vi "Interface.vi"() -> ()   [LabVIEW 2018]
uses:
  Readout Delay Charact/Readout Charact.lvclass
  CCDCamera/CCDCamera.lvclass
  Interface/Interface.lvclass
  Cooler/Cooler.lvclass
  Sync Box/Sync Box.lvclass
  State Machine/State Machine.lvclass
panel:
  in  "Trigger":u16(ring) items=["Internal", "External", "N/A", "N/A", "N/A", "N/A", "External Start"]
  in  "Vertical Clock  Amplitude":u8(ring) items=["Normal", "+1", "+2", "+3", "+4"]
  out "Readout Time (ms)":dbl=0.039386453333333335
  in  "Camera Setup":T1={"Image Name"="Image", "Image Path"="C:\\Users\\Cliente\\Desktop\\SPARC4_AC\\Imagens\\", "# Images"=0, "Exposure Time"=0.0, "Pre-amp gain"=0, "Readout Rate"=0, "Vertical Shift Speed"=3, "Acquisition Mode"=1, "Read Mode"=4, "EM Mode"=0, "EM Gain"=2, "Shutter Mode"=2, "Shutter TTL"=0, "Time to open shutter"=50, "Time to close shutter"=50, "Vertical Binning"=1, "Horizontal Binning"=1, "Initial Line"=1, "Initial Cloumn"=1, "Final Line"=1024, "Final Column"=1024, "Cooler ON/OFF"=0, "Set temperature"=20, "Number of exp"=0, "Exposições realizadas"=0, "Kinetic Serie Length"=0, "Number of Accumulations"=0, "Kinetic Cycle Time"=0, "Frame Transfer"=FALSE, "Vertical Clock  Amplitude"=0, "Trigger"=0} {"Trigger" items=["Internal", "External", "N/A", "N/A", "N/A", "N/A", "External Start"]; "Vertical Clock  Amplitude" items=["Normal", "+1", "+2", "+3", "+4"]; "Set temperature" min=0 max=0; "Cooler ON/OFF" items=["Cooler OFF", "Cooler ON"]; "Shutter TTL" items=["TTL Low", "TTl High"]; "Shutter Mode" items=["Fully Auto", "OPEN", "CLOSED"]; "EM Mode" items=["Electron Multiplying", "Conventional"]; "Read Mode" items=["Full Vertical Binning", "Multi-Track", "Random-track", "Single-Track", "Image"]; "Acquisition Mode" items=["N/A", "Single", "Accumulate", "Kinetic", "Fast Kinetic"]; "Vertical Shift Speed" items=["0.6", "1.13", "2.2", "4.33"]; "Readout Rate" items=["1 MHz", "10 MHz", "20 MHz", "30 MHz"]; "Pre-amp gain" items=["Gain 1", "Gain 2"]}
  in  "Frame Transfer":bool
  in  "Number of Accum.":u32=1 min=1
  in  "Kinetic Cycle Time":u32
  in  "Kinetic Series Length":u32=1 min=1
  out "String":string="#img      1st Time       2nd Time      3th Time      4th Time      5th Time\n------------------------------------------------------------------------\n"
  in  "Tempo de espera":u16=20
  out "Calculated Delay Series:":dbl
  in  "Address:":string="192.168.254.183"
  in  "Remote Port:":u32=2000
  in  "Stop Button":bool
  in  "Readout Charact in":refnum<class "Readout Charact.lvclass">
  in  "Vertical Binning":u16=1
  in  "Horizontal Binning":u16=1
  in  "Final Line":u16=1024
  in  "Final Column":u16=1024
  in  "Initial Cloumn":u16=1
  in  "Initial Line":u16=1
  in  "Time to open shutter":u16=50
  in  "Time to close shutter":u16=50
  in  "Shutter Mode":u8(ring)=2 items=["Fully Auto", "OPEN", "CLOSED"]
  in  "Shutter TTL":u8(ring) items=["TTL Low", "TTl High"]
  in  "Set temperature":i8=20 min=-120 max=20
  in  "Cooler ON/OFF":u16(ring) items=["Cooler OFF", "Cooler ON"]
  in  "EM Mode":u8(ring) items=["Electron Multiplying", "Conventional"]
  in  "EM Gain":u16=2 min=2 max=300
  in  "Pre-amp gain":u8(ring) items=["Gain 1", "Gain 2", "Gain 3"]
  in  "Readout Rate":u8(ring) items=["30 MHz", "20 MHz", "10 MHz", "  1 MHz"]
  in  "Vertical Shift Speed":u8(ring)=3 items=["0.6", "1.13", "2.2", "4.33"]
  in  "Acquisition Mode":u8(ring)=1 items=["N/A", "Single", "Accumulate", "Kinetic", "Fast Kinetic"]
  in  "Read Mode":u8(ring)=4 items=["Full Vertical Binning", "Multi-Track", "Random-track", "Single-Track", "Image"]
  in  "Image Name":string="CH1"
  out "Initialization":bool
  in  "Exposure Time":u32
  in  "# Images":u32=1 min=1
  out "Temperature":i16
  out "Exposing":bool
  out "% Acquired":dbl format="%#.2g"
  out "Exposições realizadas":u8(slide) max=1 scale=0.0..1.0
  in  "Abort":bool
  in  "Adquirir":bool
  in  "Stop Acq":bool
  in  "Pausar":bool
  in  "Image Path":string="C:\\Users\\observer\\Desktop\\SPARC4 Acquisition Control\\Imagens"
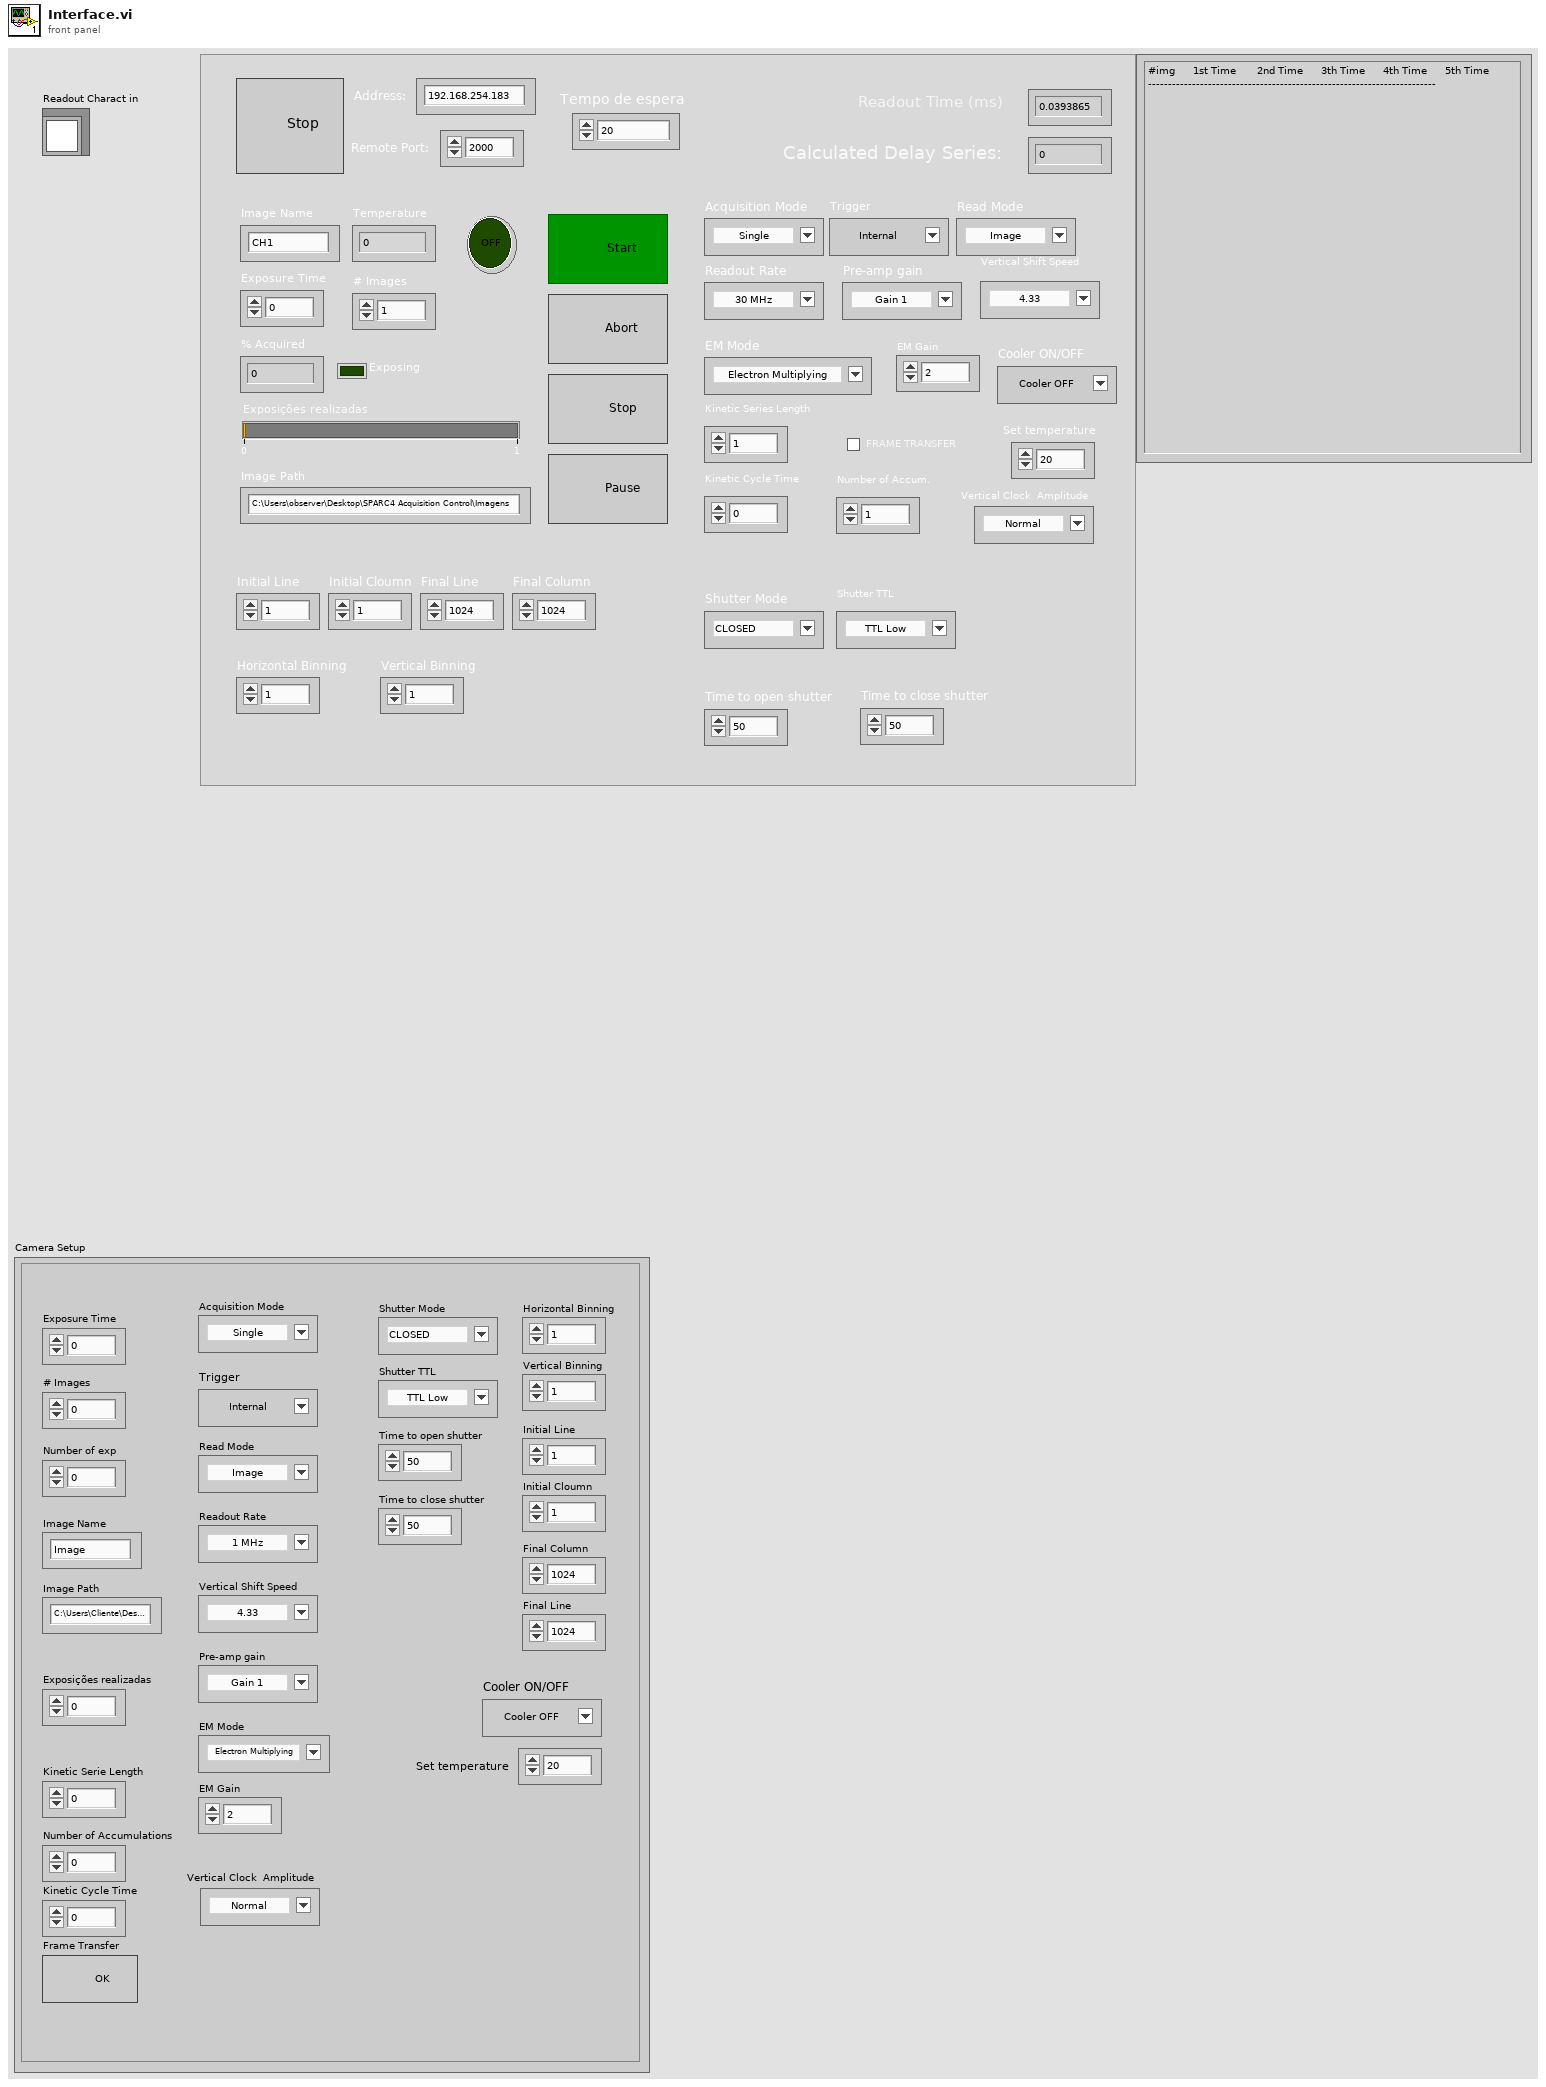
[diagram p1: front panel]
types:
  T1 = cluster{"Image Name":string, "Image Path":string, "# Images":u32, "Exposure Time":dbl, "Pre-amp gain":u8, "Readout Rate":u8, "Vertical Shift Speed":u8, "Acquisition Mode":u8, "Read Mode":u8, "EM Mode":u8, "EM Gain":u16, "Shutter Mode":u8, "Shutter TTL":u8, "Time to open shutter":u16, "Time to close shutter":u16, "Vertical Binning":u16, "Horizontal Binning":u16, "Initial Line":u16, "Initial Cloumn":u16, "Final Line":u16, "Final Column":u16, "Cooler ON/OFF":u16, "Set temperature":i8, "Number of exp":u32, "Exposições realizadas":u16, "Kinetic Serie Length":u32, "Number of Accumulations":u32, "Kinetic Cycle Time":u32, "Frame Transfer":bool, "Vertical Clock  Amplitude":u8, "Trigger":u16}
  T2 = cluster{"% Acquired":dbl, "Acquiring":bool, "Current Temperature":dbl, "Temperatue Status":string, "Min Temp":dbl, "Max Temp":dbl, "Exposições realizadas":u32, "Final Column":u16, "Final Line":u16}
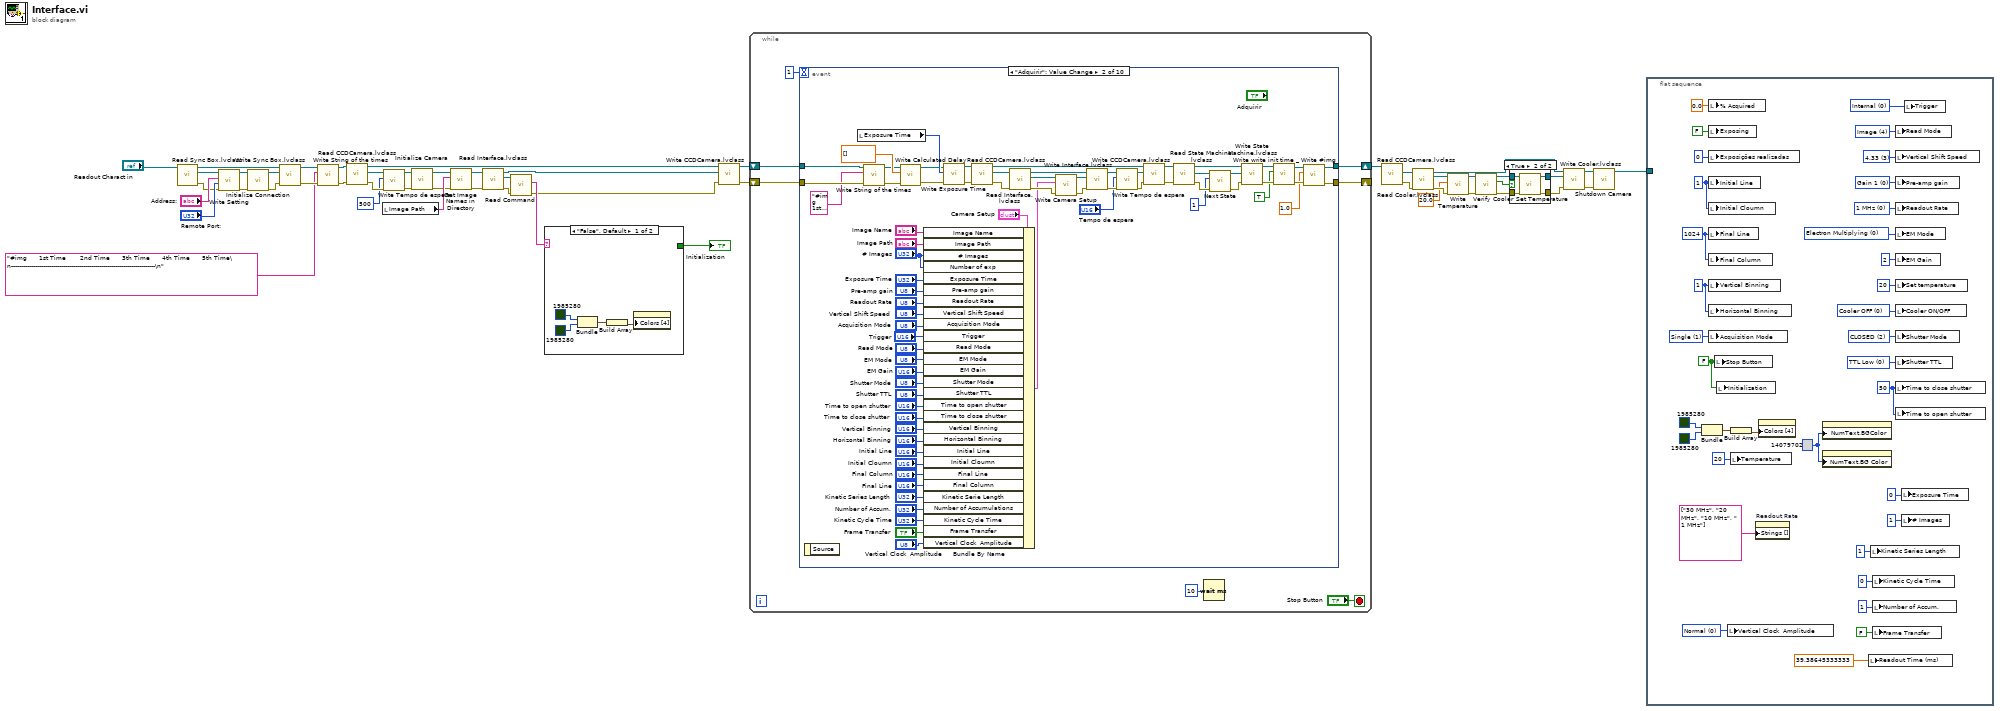
[diagram p0: block diagram]
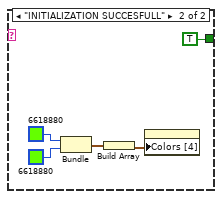
[diagram p2: hidden frame]
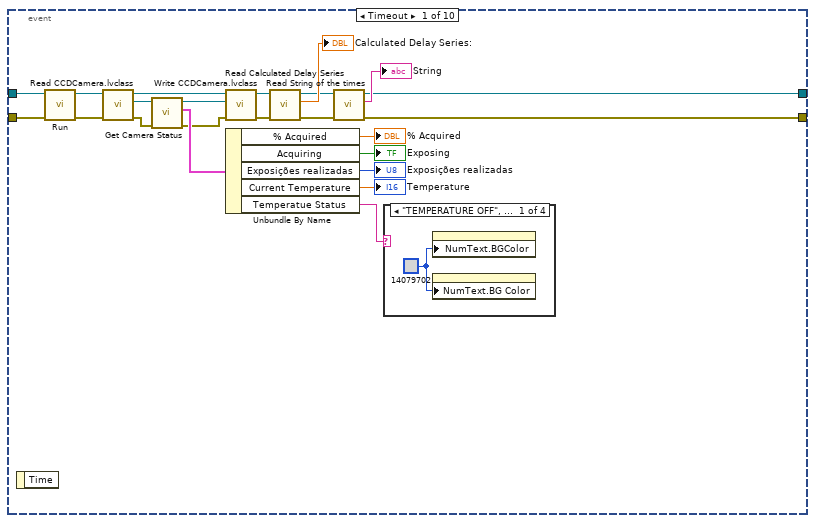
[diagram p4: hidden frame]
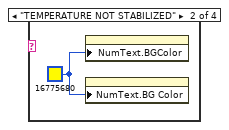
[diagram p5: hidden frame]
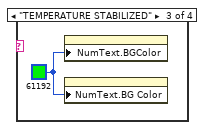
[diagram p6: hidden frame]
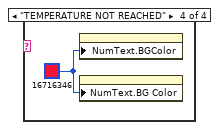
[diagram p7: hidden frame]
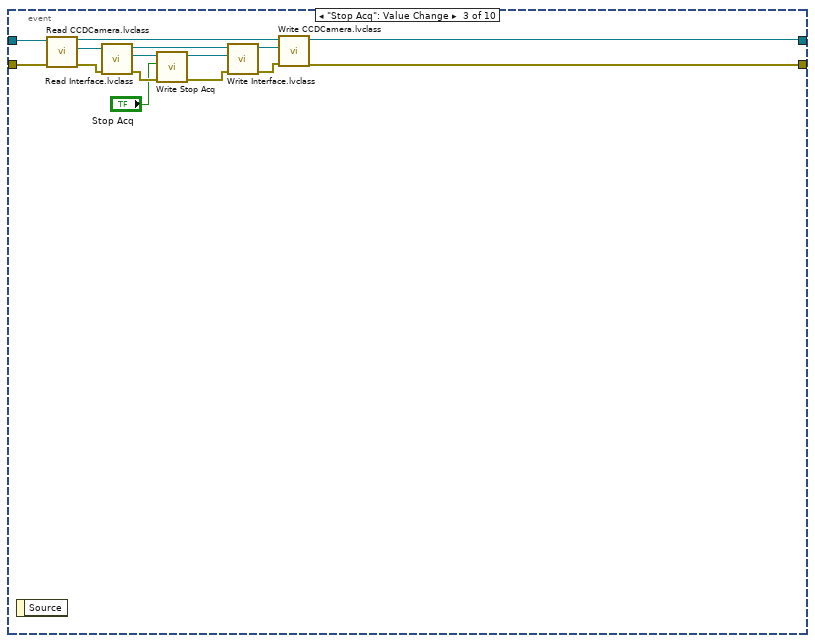
[diagram p8: hidden frame]
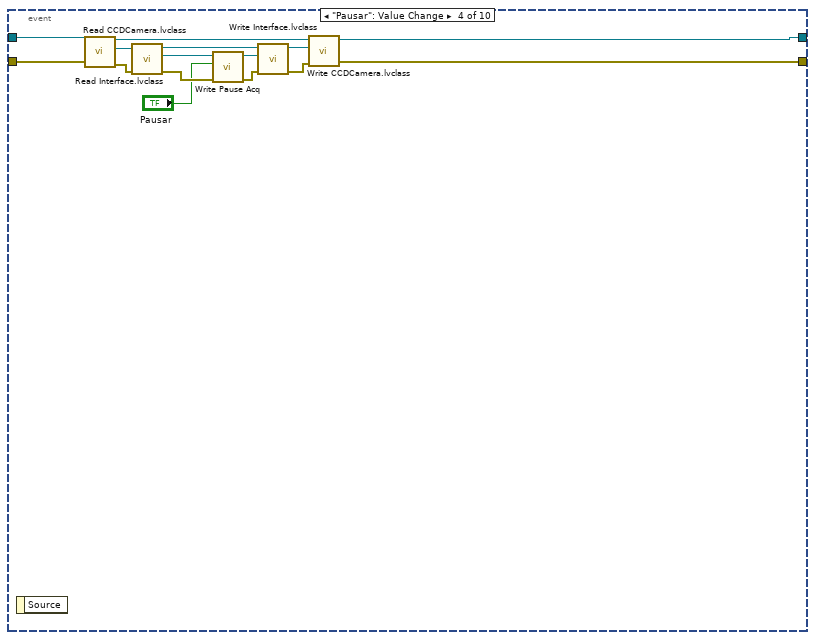
[diagram p9: hidden frame]
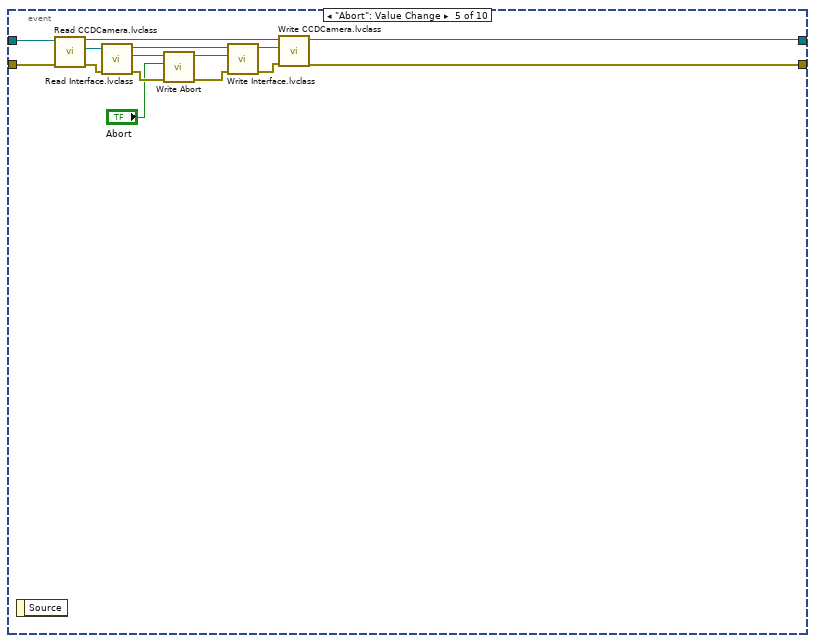
[diagram p10: hidden frame]
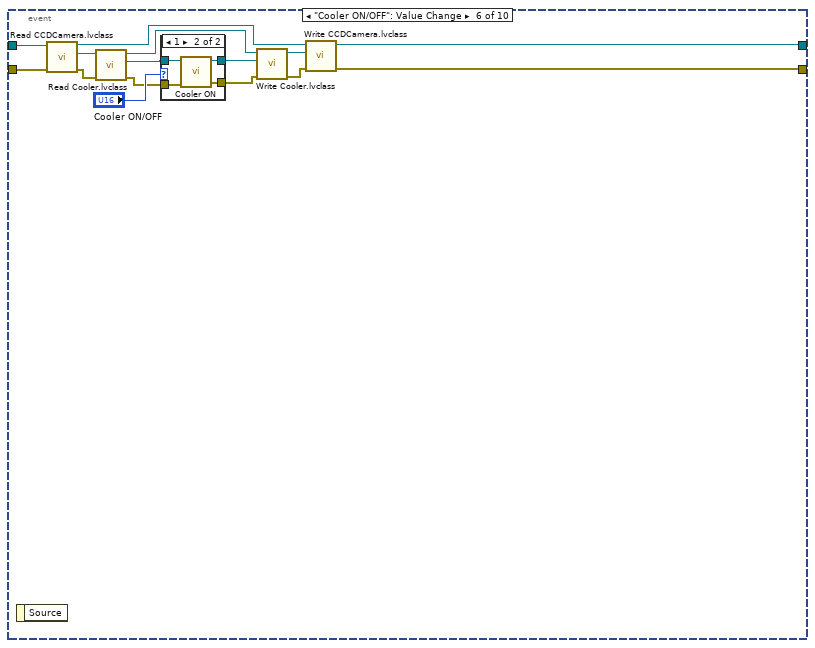
[diagram p11: hidden frame]
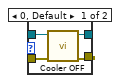
[diagram p12: hidden frame]
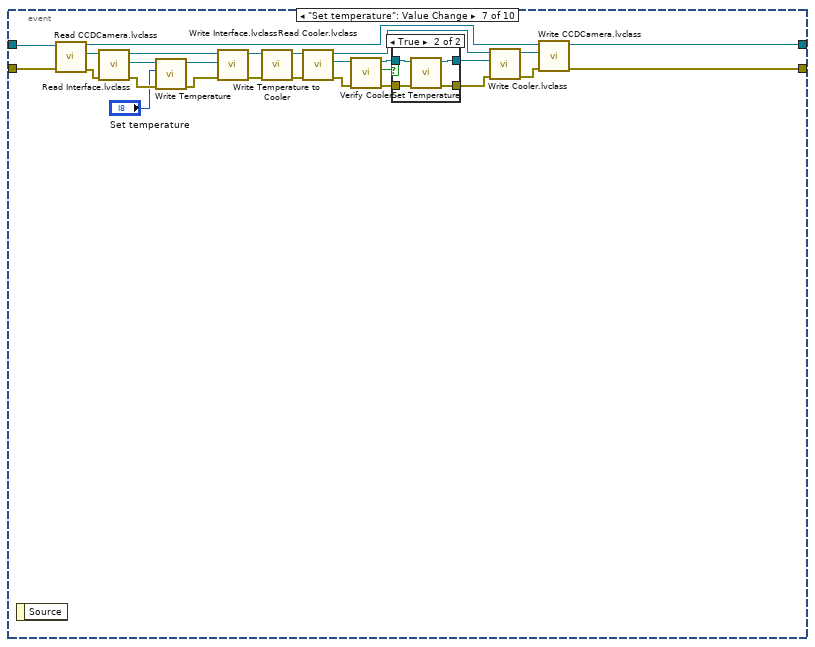
[diagram p13: hidden frame]
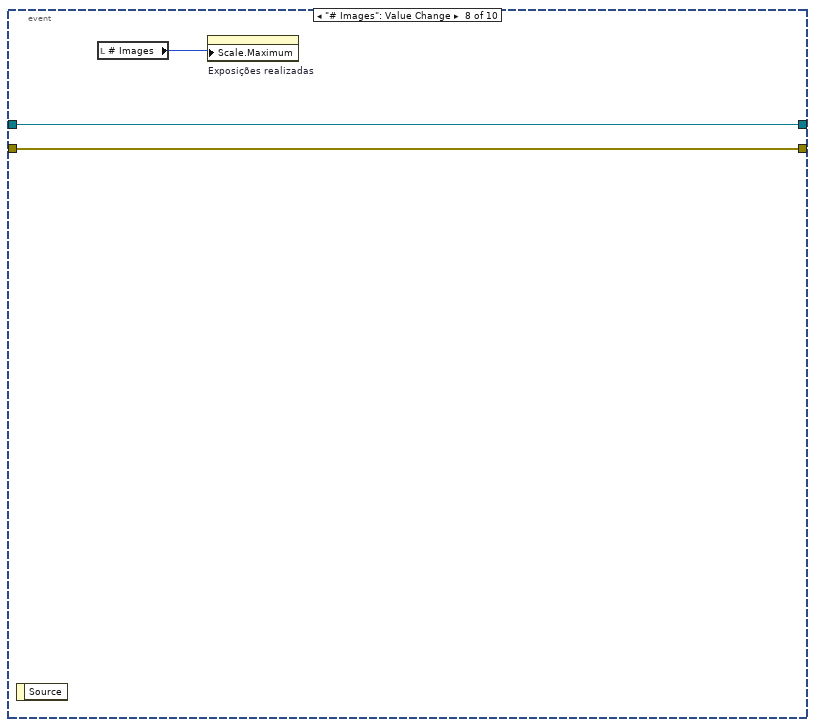
[diagram p15: hidden frame]
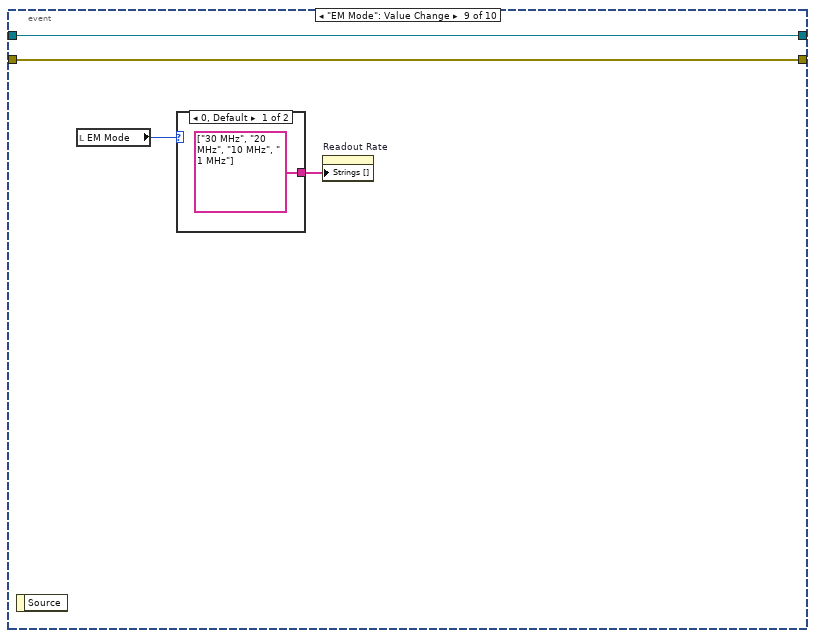
[diagram p16: hidden frame]
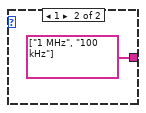
[diagram p17: hidden frame]
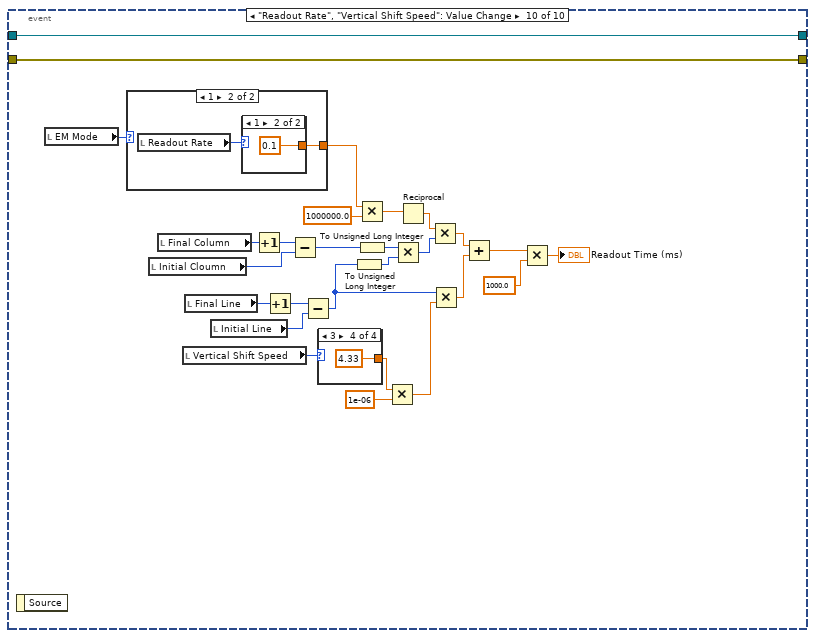
[diagram p18: hidden frame]
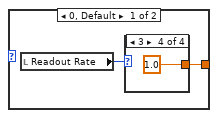
[diagram p19: hidden frame]
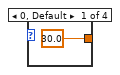
[diagram p20: hidden frame]
diagram:
  n1 = call-dynamic "Read Sync Box.lvclass.vi"("Readout Charact in"="Readout Charact in") -> ("error out"=w25:errorcluster, "Sync Box.lvclass"=w28:refnum<class "Sync Box.lvclass">, "Readout Charact out"=w24:refnum<class "Readout Charact.lvclass">)  [unwired: 8 in]
  n2 = call "Write Setting.vi"("error in (no error)"=w25, "Remote Port"="Remote Port:", "Address"="Address:", "Sync Box in"=w28) -> ("error out"=w32:errorcluster, "Sync Box out"=w31:refnum<class "Sync Box.lvclass">)  [unwired: 6 in]
  n3 = call "Initialize Connection.vi"("error in (no error)"=w32, "Sync Box in"=w31) -> ("error out"=w26:errorcluster, "Sync Box out"=w27:refnum<class "Sync Box.lvclass">)  [unwired: 7 in, 1 out]
  n4 = call-dynamic "Write Sync Box.lvclass.vi"("error in (no error)"=w26, "Sync Box.lvclass"=w27, "Readout Charact in"=w24) -> ("error out"=w12:errorcluster, "Readout Charact out"=w11:refnum<class "Readout Charact.lvclass">)  [unwired: 7 in]
  n5 = call-dynamic "Write String of the times.vi"("error in (no error)"=w12, "String of the times"="#img      1st Time       2nd Time      3th Time      4th Time      5th Time\n------------------------------------------------------------------------\n" ("String 2"), "Readout Charact in"=w11) -> ("error out"=w9:errorcluster, "Readout Charact out"=w10:refnum<class "Readout Charact.lvclass">)  [unwired: 7 in]
  n6 = call-dynamic "Read CCDCamera.lvclass.vi"("error in (no error)"=w9, "Readout Charact in"=w10) -> ("error out"=w14:errorcluster, "CCDCamera.lvclass"=w15:refnum<class "CCDCamera.lvclass">, "Readout Charact out"=w51:refnum<class "Readout Charact.lvclass">)  [unwired: 7 in]
  n7 = local read "Image Path"() -> (w3:string)
  n8 = call-dynamic "Write Tempo de espera.vi"("error in (no error)"=w14, "Tempo de espera"=500, "CCDCamera in"=w15) -> ("error out"=w17:errorcluster, "CCDCamera out"=w16:refnum<class "CCDCamera.lvclass">)  [unwired: 7 in]
  n9 = call "Initialize Camera.vi"("error in (no error)"=w17, "CCDCamera in"=w16) -> ("error out"=w2:errorcluster, "CCDCamera out"=w1:refnum<class "CCDCamera.lvclass">)  [unwired: 8 in]
  n10 = call "Get Image Names in Directory.vi"("error in (no error)"=w2, "Image Path"=w3, "CCDCamera in"=w1) -> ("error out"=w4:errorcluster, "CCDCamera out"=w5:refnum<class "CCDCamera.lvclass">)  [unwired: 7 in]
  n11 = call-dynamic "Read Interface.lvclass.vi"("error in (no error)"=w4, "CCDCamera in"=w5) -> ("error out"=w21:errorcluster, "Interface.lvclass"=w22:refnum<class "Interface.lvclass">, "CCDCamera out"=w6:refnum<class "CCDCamera.lvclass">)  [unwired: 7 in]
  n12 = call "Read Command.vi"("error in (no error)"=w21, "Interface in"=w22) -> ("error out"=w7:errorcluster, "Command"=w20:string)  [unwired: 7 in, 1 out]
  n13 = case shown="\"False\", Default" w20 {
    tunnel: [_ TRUE ("Initialization")] -> w19
    frame "False", Default {
      n14 = Bundle(u32 1985280, u32 1985280) -> (w55:cluster{u32, u32})  [unwired: 1 in]
      n15 = Build Array(w55) -> (w54:cluster{u32, u32}[])
      n16 = property on="Initialization" class="Bool (strict)"("Colors [4]"=w54) -> ()  [unwired: 2 in, 2 out]
    }
    frame "INITIALIZATION SUCCESFULL" {
      n17 = Bundle(u32 6618880, u32 6618880) -> (w59:cluster{u32, u32})  [unwired: 1 in]
      n18 = Build Array(w59) -> (w56:cluster{u32, u32}[])
      n19 = property on="Initialization" class="Bool (strict)"("Colors [4]"=w56) -> ()  [unwired: 2 in, 2 out]
    }
  }
  "Initialization" <- w19
  n20 = call-dynamic "Write CCDCamera.lvclass.vi"("error in (no error)"=w7, "CCDCamera.lvclass"=w6, "Readout Charact in"=w51) -> ("error out"=w49:errorcluster, "Readout Charact out"=w50:refnum<class "Readout Charact.lvclass">)  [unwired: 7 in]
  n21 = while {
    shift-right: [w63] -> w33
    shift-left: w50 -> [w65]
    shift-right: [w62] -> _
    shift-left: w49 -> [w64]
    stop <- "Stop Button" stop-if-true
    n22 = event shown="[1] \"Adquirir\": Value Change" {
      selector: _ -> [_ _ _ _ _ _ _ _ _ _]
      dyn-events: _ -> [_ _ _ _ _ _ _ _ _ _]
      timeout: 1 -> [_ _ _ _ _ _ _ _ _ _]
      tunnel: w65 -> [w77 w114 w177 w187 w202 w222 w255 w266 w270 w299]
      tunnel: w64 -> [w76 w113 w178 w186 w201 w223 w254 w265 w271 w300]
      tunnel: [w68 w111 w166 w185 w200 w210 w253 w266 w270 w299] -> w63
      tunnel: [w69 w112 w165 w184 w199 w209 w252 w265 w271 w300] -> w62
      event Timeout {
        n23 = event-data() -> ()  [unwired: 1 in, 1 out]
        n24 = call "Run.vi"("error in (no error)"=w76, "Readout Charact in"=w77) -> ("error out"=w79:errorcluster, "Readout Charact out"=w78:refnum<class "Readout Charact.lvclass">)  [unwired: 8 in]
        n25 = call-dynamic "Read CCDCamera.lvclass.vi"("error in (no error)"=w79, "Readout Charact in"=w78) -> ("error out"=w89:errorcluster, "CCDCamera.lvclass"=w90:refnum<class "CCDCamera.lvclass">, "Readout Charact out"=w80:refnum<class "Readout Charact.lvclass">)  [unwired: 7 in]
        n26 = call "Get Camera Status.vi"("error in (no error)"=w89, "CCDCamera in"=w90) -> ("error out"=w82:errorcluster, "Camera Status"=w87:T2, "CCDCamera out"=w81:refnum<class "CCDCamera.lvclass">)  [unwired: 7 in]
        n27 = call-dynamic "Write CCDCamera.lvclass.vi"("error in (no error)"=w82, "CCDCamera.lvclass"=w81, "Readout Charact in"=w80) -> ("error out"=w74:errorcluster, "Readout Charact out"=w73:refnum<class "Readout Charact.lvclass">)  [unwired: 7 in]
        n28 = Unbundle By Name(w87) -> ("% Acquired"=→"% Acquired":dbl, "Acquiring"=→"Exposing":bool, "Exposições realizadas"=→"Exposições realizadas":u32, "Current Temperature"=→"Temperature":dbl, "Temperatue Status"=w88:string)
        n29 = call-dynamic "Read Calculated Delay Series.vi"("error in (no error)"=w74, "Readout Charact in"=w73) -> ("error out"=w72:errorcluster, "Calculated Delay Series"=→"Calculated Delay Series:":dbl, "Readout Charact out"=w71:refnum<class "Readout Charact.lvclass">)  [unwired: 7 in]
        n30 = call-dynamic "Read String of the times.vi"("error in (no error)"=w72, "Readout Charact in"=w71) -> ("error out"=w69:errorcluster, "String of the times"=→"String":string, "Readout Charact out"=w68:refnum<class "Readout Charact.lvclass">)  [unwired: 7 in]
        n31 = case shown="\"TEMPERATURE OFF\", Default" w88 {
          frame "TEMPERATURE OFF", Default {
            w91 = u32 14079702
            n32 = property on="Temperature" class="DigNum (strict)"("NumText.BGColor"=w91) -> ()  [unwired: 2 in, 2 out]
            n33 = property on="Temperature" class="DigNum (strict)"("NumText.BG Color"=w91) -> ()  [unwired: 2 in, 2 out]
          }
          frame "TEMPERATURE NOT STABILIZED" {
            w92 = u32 16775680
            n34 = property on="Temperature" class="DigNum (strict)"("NumText.BGColor"=w92) -> ()  [unwired: 2 in, 2 out]
            n35 = property on="Temperature" class="DigNum (strict)"("NumText.BG Color"=w92) -> ()  [unwired: 2 in, 2 out]
          }
          frame "TEMPERATURE STABILIZED" {
            w93 = u32 61192
            n36 = property on="Temperature" class="DigNum (strict)"("NumText.BGColor"=w93) -> ()  [unwired: 2 in, 2 out]
            n37 = property on="Temperature" class="DigNum (strict)"("NumText.BG Color"=w93) -> ()  [unwired: 2 in, 2 out]
          }
          frame "TEMPERATURE NOT REACHED" {
            w94 = u32 16716346
            n38 = property on="Temperature" class="DigNum (strict)"("NumText.BGColor"=w94) -> ()  [unwired: 2 in, 2 out]
            n39 = property on="Temperature" class="DigNum (strict)"("NumText.BG Color"=w94) -> ()  [unwired: 2 in, 2 out]
          }
        }
      }
      event "Adquirir": Value Change {
        n40 = event-data() -> ()  [unwired: 1 in, 1 out]
        n41 = local read "Exposure Time"() -> (w125:u32)
        n42 = call-dynamic "Write String of the times.vi"("error in (no error)"=w113, "String of the times"="#img      1st Time       2nd Time      3th Time      4th Time      5th Time\n------------------------------------------------------------------------\n" ("String 2"), "Readout Charact in"=w114) -> ("error out"=w116:errorcluster, "Readout Charact out"=w115:refnum<class "Readout Charact.lvclass">)  [unwired: 7 in]
        n43 = call-dynamic "Write Calculated Delay.vi"("error in (no error)"=w116, "Calculated Delay"=dbl[] [], "Readout Charact in"=w115) -> ("error out"=w118:errorcluster, "Readout Charact out"=w119:refnum<class "Readout Charact.lvclass">)  [unwired: 7 in]
        n44 = Bundle By Name(cluster="Camera Setup", "Image Name"="Image Name", "Image Path"="Image Path", "# Images"="# Images", "Number of exp"="# Images", "Exposure Time"="Exposure Time", "Pre-amp gain"="Pre-amp gain", "Readout Rate"="Readout Rate", "Vertical Shift Speed"="Vertical Shift Speed", "Acquisition Mode"="Acquisition Mode", "Trigger"="Trigger", "Read Mode"="Read Mode", "EM Mode"="EM Mode", "EM Gain"="EM Gain", "Shutter Mode"="Shutter Mode", "Shutter TTL"="Shutter TTL", "Time to open shutter"="Time to open shutter", "Time to close shutter"="Time to close shutter", "Vertical Binning"="Vertical Binning", "Horizontal Binning"="Horizontal Binning", "Initial Line"="Initial Line", "Initial Cloumn"="Initial Cloumn", "Final Line"="Final Line", "Final Column"="Final Column", "Kinetic Serie Length"="Kinetic Series Length", "Number of Accumulations"="Number of Accum.", "Kinetic Cycle Time"="Kinetic Cycle Time", "Frame Transfer"="Frame Transfer", "Vertical Clock  Amplitude"="Vertical Clock  Amplitude") -> (w156:T1)
        n45 = call-dynamic "Write Exposure Time.vi"("error in (no error)"=w118, "Exposure Time"=w125, "Readout Charact in"=w119) -> ("error out"=w123:errorcluster, "Readout Charact out"=w124:refnum<class "Readout Charact.lvclass">)  [unwired: 7 in]
        n46 = call-dynamic "Read CCDCamera.lvclass.vi"("error in (no error)"=w123, "Readout Charact in"=w124) -> ("error out"=w162:errorcluster, "CCDCamera.lvclass"=w163:refnum<class "CCDCamera.lvclass">, "Readout Charact out"=w134:refnum<class "Readout Charact.lvclass">)  [unwired: 7 in]
        n47 = call-dynamic "Read Interface.lvclass.vi"("error in (no error)"=w162, "CCDCamera in"=w163) -> ("error out"=w160:errorcluster, "Interface.lvclass"=w161:refnum<class "Interface.lvclass">, "CCDCamera out"=w157:refnum<class "CCDCamera.lvclass">)  [unwired: 7 in]
        n48 = call "Write Camera Setup.vi"("error in (no error)"=w160, "Camera Setup"=w156, "Interface in"=w161) -> ("error out"=w159:errorcluster, "Interface out"=w158:refnum<class "Interface.lvclass">)  [unwired: 7 in]
        n49 = call-dynamic "Write Interface.lvclass.vi"("error in (no error)"=w159, "Interface.lvclass"=w158, "CCDCamera in"=w157) -> ("error out"=w107:errorcluster, "CCDCamera out"=w106:refnum<class "CCDCamera.lvclass">)  [unwired: 7 in]
        n50 = call-dynamic "Write Tempo de espera.vi"("error in (no error)"=w107, "Tempo de espera"="Tempo de espera", "CCDCamera in"=w106) -> ("error out"=w104:errorcluster, "CCDCamera out"=w105:refnum<class "CCDCamera.lvclass">)  [unwired: 7 in]
        n51 = call-dynamic "Write CCDCamera.lvclass.vi"("error in (no error)"=w104, "CCDCamera.lvclass"=w105, "Readout Charact in"=w134) -> ("error out"=w133:errorcluster, "Readout Charact out"=w132:refnum<class "Readout Charact.lvclass">)  [unwired: 7 in]
        n52 = call-dynamic "Read State Machine.lvclass.vi"("error in (no error)"=w133, "Readout Charact in"=w132) -> ("error out"=w130:errorcluster, "State Machine.lvclass"=w131:refnum<class "State Machine.lvclass">, "Readout Charact out"=w126:refnum<class "Readout Charact.lvclass">)  [unwired: 7 in]
        n53 = call "Next State.vi"("error in (no error)"=w130, "New_State"=1, "State Machine in"=w131) -> ("error out"=w128:errorcluster, "State Machine out"=w127:refnum<class "State Machine.lvclass">)  [unwired: 7 in]
        n54 = call-dynamic "Write State Machine.lvclass.vi"("error in (no error)"=w128, "State Machine.lvclass"=w127, "Readout Charact in"=w126) -> ("error out"=w121:errorcluster, "Readout Charact out"=w122:refnum<class "Readout Charact.lvclass">)  [unwired: 7 in]
        n55 = call-dynamic "Write write init time _.vi"("error in (no error)"=w121, "write init time ?"=TRUE, "Readout Charact in"=w122) -> ("error out"=w109:errorcluster, "Readout Charact out"=w110:refnum<class "Readout Charact.lvclass">)  [unwired: 7 in]
        n56 = call-dynamic "Write #img.vi"("error in (no error)"=w109, "#img"=1.0, "Readout Charact in"=w110) -> ("error out"=w112:errorcluster, "Readout Charact out"=w111:refnum<class "Readout Charact.lvclass">)  [unwired: 7 in]
      }
      event "Stop Acq": Value Change {
        n57 = event-data() -> ()  [unwired: 1 in, 1 out]
        n58 = call-dynamic "Read CCDCamera.lvclass.vi"("error in (no error)"=w178, "Readout Charact in"=w177) -> ("error out"=w175:errorcluster, "CCDCamera.lvclass"=w176:refnum<class "CCDCamera.lvclass">, "Readout Charact out"=w167:refnum<class "Readout Charact.lvclass">)  [unwired: 7 in]
        n59 = call-dynamic "Read Interface.lvclass.vi"("error in (no error)"=w175, "CCDCamera in"=w176) -> ("error out"=w173:errorcluster, "Interface.lvclass"=w174:refnum<class "Interface.lvclass">, "CCDCamera out"=w170:refnum<class "CCDCamera.lvclass">)  [unwired: 7 in]
        n60 = call-dynamic "Write Stop Acq.vi"("error in (no error)"=w173, "Stop Acq"="Stop Acq", "Interface in"=w174) -> ("error out"=w172:errorcluster, "Interface out"=w171:refnum<class "Interface.lvclass">)  [unwired: 7 in]
        n61 = call-dynamic "Write Interface.lvclass.vi"("error in (no error)"=w172, "Interface.lvclass"=w171, "CCDCamera in"=w170) -> ("error out"=w169:errorcluster, "CCDCamera out"=w168:refnum<class "CCDCamera.lvclass">)  [unwired: 7 in]
        n62 = call-dynamic "Write CCDCamera.lvclass.vi"("error in (no error)"=w169, "CCDCamera.lvclass"=w168, "Readout Charact in"=w167) -> ("error out"=w165:errorcluster, "Readout Charact out"=w166:refnum<class "Readout Charact.lvclass">)  [unwired: 7 in]
      }
      event "Pausar": Value Change {
        n63 = event-data() -> ()  [unwired: 1 in, 1 out]
        n64 = call-dynamic "Read CCDCamera.lvclass.vi"("error in (no error)"=w186, "Readout Charact in"=w187) -> ("error out"=w192:errorcluster, "CCDCamera.lvclass"=w193:refnum<class "CCDCamera.lvclass">, "Readout Charact out"=w188:refnum<class "Readout Charact.lvclass">)  [unwired: 7 in]
        n65 = call-dynamic "Read Interface.lvclass.vi"("error in (no error)"=w192, "CCDCamera in"=w193) -> ("error out"=w180:errorcluster, "Interface.lvclass"=w183:refnum<class "Interface.lvclass">, "CCDCamera out"=w191:refnum<class "CCDCamera.lvclass">)  [unwired: 7 in]
        n66 = call-dynamic "Write Pause Acq.vi"("error in (no error)"=w180, "Pause Acq"="Pausar", "Interface in"=w183) -> ("error out"=w181:errorcluster, "Interface out"=w182:refnum<class "Interface.lvclass">)  [unwired: 7 in]
        n67 = call-dynamic "Write Interface.lvclass.vi"("error in (no error)"=w181, "Interface.lvclass"=w182, "CCDCamera in"=w191) -> ("error out"=w190:errorcluster, "CCDCamera out"=w189:refnum<class "CCDCamera.lvclass">)  [unwired: 7 in]
        n68 = call-dynamic "Write CCDCamera.lvclass.vi"("error in (no error)"=w190, "CCDCamera.lvclass"=w189, "Readout Charact in"=w188) -> ("error out"=w184:errorcluster, "Readout Charact out"=w185:refnum<class "Readout Charact.lvclass">)  [unwired: 7 in]
      }
      event "Abort": Value Change {
        n69 = event-data() -> ()  [unwired: 1 in, 1 out]
        n70 = call-dynamic "Read CCDCamera.lvclass.vi"("error in (no error)"=w201, "Readout Charact in"=w202) -> ("error out"=w207:errorcluster, "CCDCamera.lvclass"=w208:refnum<class "CCDCamera.lvclass">, "Readout Charact out"=w203:refnum<class "Readout Charact.lvclass">)  [unwired: 7 in]
        n71 = call-dynamic "Read Interface.lvclass.vi"("error in (no error)"=w207, "CCDCamera in"=w208) -> ("error out"=w195:errorcluster, "Interface.lvclass"=w196:refnum<class "Interface.lvclass">, "CCDCamera out"=w206:refnum<class "CCDCamera.lvclass">)  [unwired: 7 in]
        n72 = call-dynamic "Write Abort.vi"("error in (no error)"=w195, "Abort"="Abort", "Interface in"=w196) -> ("error out"=w197:errorcluster, "Interface out"=w198:refnum<class "Interface.lvclass">)  [unwired: 7 in]
        n73 = call-dynamic "Write Interface.lvclass.vi"("error in (no error)"=w197, "Interface.lvclass"=w198, "CCDCamera in"=w206) -> ("error out"=w205:errorcluster, "CCDCamera out"=w204:refnum<class "CCDCamera.lvclass">)  [unwired: 7 in]
        n74 = call-dynamic "Write CCDCamera.lvclass.vi"("error in (no error)"=w205, "CCDCamera.lvclass"=w204, "Readout Charact in"=w203) -> ("error out"=w199:errorcluster, "Readout Charact out"=w200:refnum<class "Readout Charact.lvclass">)  [unwired: 7 in]
      }
      event "Cooler ON/OFF": Value Change {
        n75 = event-data() -> ()  [unwired: 1 in, 1 out]
        n76 = call-dynamic "Read CCDCamera.lvclass.vi"("error in (no error)"=w223, "Readout Charact in"=w222) -> ("error out"=w220:errorcluster, "CCDCamera.lvclass"=w221:refnum<class "CCDCamera.lvclass">, "Readout Charact out"=w211:refnum<class "Readout Charact.lvclass">)  [unwired: 7 in]
        n77 = call-dynamic "Read Cooler.lvclass.vi"("error in (no error)"=w220, "CCDCamera in"=w221) -> ("error out"=w217:errorcluster, "Cooler.lvclass"=w218:refnum<class "Cooler.lvclass">, "CCDCamera out"=w214:refnum<class "CCDCamera.lvclass">)  [unwired: 7 in]
        n78 = case shown="1" "Cooler ON/OFF" {
          tunnel: w218 -> [w227 w229]
          tunnel: w217 -> [w226 w228]
          tunnel: [w225 w230] -> w215
          tunnel: [w224 w231] -> w216
          frame 0, Default {
            n79 = call "Cooler OFF.vi"("error in (no error)"=w226, "Cooler in"=w227) -> ("error out"=w225:errorcluster, "Cooler out"=w224:refnum<class "Cooler.lvclass">)  [unwired: 8 in]
          }
          frame 1 {
            n80 = call "Cooler ON.vi"("error in (no error)"=w228, "Cooler in"=w229) -> ("error out"=w230:errorcluster, "Cooler out"=w231:refnum<class "Cooler.lvclass">)  [unwired: 8 in]
          }
        }
        n81 = call-dynamic "Write Cooler.lvclass.vi"("error in (no error)"=w215, "Cooler.lvclass"=w216, "CCDCamera in"=w214) -> ("error out"=w212:errorcluster, "CCDCamera out"=w213:refnum<class "CCDCamera.lvclass">)  [unwired: 7 in]
        n82 = call-dynamic "Write CCDCamera.lvclass.vi"("error in (no error)"=w212, "CCDCamera.lvclass"=w213, "Readout Charact in"=w211) -> ("error out"=w209:errorcluster, "Readout Charact out"=w210:refnum<class "Readout Charact.lvclass">)  [unwired: 7 in]
      }
      event "Set temperature": Value Change {
        n83 = event-data() -> ()  [unwired: 1 in, 1 out]
        n84 = call-dynamic "Read CCDCamera.lvclass.vi"("error in (no error)"=w254, "Readout Charact in"=w255) -> ("error out"=w242:errorcluster, "CCDCamera.lvclass"=w243:refnum<class "CCDCamera.lvclass">, "Readout Charact out"=w256:refnum<class "Readout Charact.lvclass">)  [unwired: 7 in]
        n85 = call-dynamic "Read Interface.lvclass.vi"("error in (no error)"=w242, "CCDCamera in"=w243) -> ("error out"=w238:errorcluster, "Interface.lvclass"=w241:refnum<class "Interface.lvclass">, "CCDCamera out"=w239:refnum<class "CCDCamera.lvclass">)  [unwired: 7 in]
        n86 = call-dynamic "Write Temperature.vi"("error in (no error)"=w238, "Temperature"="Set temperature", "Interface in"=w241) -> ("error out"=w237:errorcluster, "Interface out"=w240:refnum<class "Interface.lvclass">)  [unwired: 7 in]
        n87 = call-dynamic "Write Interface.lvclass.vi"("error in (no error)"=w237, "Interface.lvclass"=w240, "CCDCamera in"=w239) -> ("error out"=w235:errorcluster, "CCDCamera out"=w234:refnum<class "CCDCamera.lvclass">)  [unwired: 7 in]
        n88 = call "Write Temperature to Cooler.vi"("error in (no error)"=w235, "CCDCamera in"=w234) -> ("error out"=w232:errorcluster, "CCDCamera out"=w233:refnum<class "CCDCamera.lvclass">)  [unwired: 8 in]
        n89 = call-dynamic "Read Cooler.lvclass.vi"("error in (no error)"=w232, "CCDCamera in"=w233) -> ("error out"=w249:errorcluster, "Cooler.lvclass"=w250:refnum<class "Cooler.lvclass">, "CCDCamera out"=w258:refnum<class "CCDCamera.lvclass">)  [unwired: 7 in]
        n90 = call "Verify Cooler.vi"("error in (no error)"=w249, "Cooler in"=w250) -> ("error out"=w247:errorcluster, "coolerStatus"=w246:bool, "Cooler out"=w248:refnum<class "Cooler.lvclass">)  [unwired: 7 in]
        n91 = case shown="True" w246 {
          tunnel: w248 -> [w260 w264]
          tunnel: [w260 w263] -> w245
          tunnel: [w259 w262] -> w244
          tunnel: w247 -> [w259 w261]
          frame False {
          }
          frame True {
            n92 = call "Set Temperature.vi"("error in (no error)"=w261, "Cooler in"=w264) -> ("error out"=w262:errorcluster, "Cooler out"=w263:refnum<class "Cooler.lvclass">)  [unwired: 8 in]
          }
        }
        n93 = call-dynamic "Write Cooler.lvclass.vi"("error in (no error)"=w244, "Cooler.lvclass"=w245, "CCDCamera in"=w258) -> ("error out"=w251:errorcluster, "CCDCamera out"=w257:refnum<class "CCDCamera.lvclass">)  [unwired: 7 in]
        n94 = call-dynamic "Write CCDCamera.lvclass.vi"("error in (no error)"=w251, "CCDCamera.lvclass"=w257, "Readout Charact in"=w256) -> ("error out"=w252:errorcluster, "Readout Charact out"=w253:refnum<class "Readout Charact.lvclass">)  [unwired: 7 in]
      }
      event "# Images": Value Change {
        n95 = event-data() -> ()  [unwired: 1 in, 1 out]
        n96 = local read "# Images"() -> (w267:u32)
        n97 = property on="Exposições realizadas" class="Slide (strict)"("Scale.Maximum"=w267) -> ()  [unwired: 2 in, 2 out]
      }
      event "EM Mode": Value Change {
        n98 = event-data() -> ()  [unwired: 1 in, 1 out]
        n99 = local read "EM Mode"() -> (w268:u8)
        n100 = case shown="0, Default" w268 {
          tunnel: [string[] ["30 MHz", "20 MHz", "10 MHz", "  1 MHz"] ("Strings []") string[] ["1 MHz", "100 kHz"] ("Strings []")] -> w269
          frame 0, Default {
          }
          frame 1 {
          }
        }
        n101 = property on="Readout Rate" class="Ring (strict)"("Strings []"=w269) -> ()  [unwired: 2 in, 2 out]
      }
      event "Readout Rate", "Vertical Shift Speed": Value Change {
        n102 = event-data() -> ()  [unwired: 1 in, 1 out]
        n103 = local read "EM Mode"() -> (w286:u8)
        n104 = case shown="1" w286 {
          tunnel: [w301 w307] -> w285
          frame 0, Default {
            n105 = local read "Readout Rate"() -> (w302:u8)
            n106 = case shown="3" w302 {
              tunnel: [30.0 20.0 10.0 1.0] -> w301
              frame 0, Default {
              }
              frame 1 {
              }
              frame 2 {
              }
              frame 3 {
              }
            }
          }
          frame 1 {
            n107 = local read "Readout Rate"() -> (w308:u8)
            n108 = case shown="1" w308 {
              tunnel: [1.0 0.1] -> w307
              frame 0, Default {
              }
              frame 1 {
              }
            }
          }
        }
        n109 = local read "Initial Cloumn"() -> (w281:u16)
        n110 = local read "Final Column"() -> (w283:u16)
        n111 = local read "Vertical Shift Speed"() -> (w298:u8)
        n112 = local read "Final Line"() -> (w284:u16)
        n113 = local read "Initial Line"() -> (w279:u16)
        n114 = Increment(x=w283) -> (x+1=w282:u16)
        n115 = Increment(x=w284) -> (x+1=w280:u16)
        n116 = Subtract(x=w282, y=w281) -> (x-y=w276:u16)
        n117 = Subtract(x=w280, y=w279) -> (x-y=w275:u16)
        n118 = case shown="3" w298 {
          tunnel: [0.6 1.13 2.2 4.33] -> w297
          frame 0, Default {
          }
          frame 1 {
          }
          frame 2 {
          }
          frame 3 {
          }
        }
        n119 = To Unsigned Long Integer(number=w275) -> (unsigned 32bit integer=w278:u32)
        n120 = Multiply(x=w285, y=1000000.0) -> (x*y=w294:dbl)
        n121 = To Unsigned Long Integer(number=w276) -> (unsigned 32bit integer=w277:u32)
        n122 = Multiply(x=w297, y=1e-06) -> (x*y=w289:dbl)
        n123 = Multiply(x=w277, y=w278) -> (x*y=w292:u32)
        n124 = Reciprocal(x=w294) -> (1/x=w293:dbl)
        n125 = Multiply(x=w293, y=w292) -> (x*y=w291:dbl)
        n126 = Multiply(x=w275, y=w289) -> (x*y=w290:dbl)
        n127 = Add(x=w291, y=w290) -> (x+y=w288:dbl)
        n128 = Multiply(x=w288, y=1000.0) -> (x*y=→"Readout Time (ms)":dbl)
      }
    }
    n129 = Wait (ms)(milliseconds to wait=u32 10) -> ()  [unwired: 1 out]
  }
  n130 = call-dynamic "Read CCDCamera.lvclass.vi"("Readout Charact in"=w33) -> ("error out"=w34:errorcluster, "CCDCamera.lvclass"=w35:refnum<class "CCDCamera.lvclass">)  [unwired: 8 in, 1 out]
  n131 = call-dynamic "Read Cooler.lvclass.vi"("error in (no error)"=w34, "CCDCamera in"=w35) -> ("error out"=w45:errorcluster, "Cooler.lvclass"=w44:refnum<class "Cooler.lvclass">, "CCDCamera out"=w48:refnum<class "CCDCamera.lvclass">)  [unwired: 7 in]
  n132 = call-dynamic "Write Temperature.vi"("error in (no error)"=w45, "Temperature"=20.0, "Cooler in"=w44) -> ("error out"=w47:errorcluster, "Cooler out"=w46:refnum<class "Cooler.lvclass">)  [unwired: 7 in]
  n133 = call "Verify Cooler.vi"("error in (no error)"=w47, "Cooler in"=w46) -> ("error out"=w41:errorcluster, "coolerStatus"=w39:bool, "Cooler out"=w40:refnum<class "Cooler.lvclass">)  [unwired: 7 in]
  n134 = case shown="True" w39 {
    tunnel: w40 -> [w316 w320]
    tunnel: [w316 w319] -> w42
    tunnel: w41 -> [w315 w318]
    tunnel: [w315 w317] -> w43
    frame False {
    }
    frame True {
      n135 = call "Set Temperature.vi"("error in (no error)"=w318, "Cooler in"=w320) -> ("error out"=w317:errorcluster, "Cooler out"=w319:refnum<class "Cooler.lvclass">)  [unwired: 8 in]
    }
  }
  n136 = call-dynamic "Write Cooler.lvclass.vi"("error in (no error)"=w43, "Cooler.lvclass"=w42, "CCDCamera in"=w48) -> ("error out"=w38:errorcluster, "CCDCamera out"=w37:refnum<class "CCDCamera.lvclass">)  [unwired: 7 in]
  n137 = call "Shutdown Camera.vi"("error in (no error)"=w38, "CCDCamera in"=w37) -> ("CCDCamera out"=w18:refnum<class "CCDCamera.lvclass">)  [unwired: 8 in, 1 out]
  n138 = flat-sequence {
    tunnel: w18 -> [_]
    frame #0 {
      w322 = u8 0 items=["Normal", "+1", "+2", "+3", "+4"] ("Vertical Clock  Amplitude")
      w331 = u32 14079702
      w337 = FALSE ("Stop Button")
      w338 = u16 50 ("Time to close shutter")
      w339 = u8 0 items=["TTL Low", "TTl High"] ("Shutter TTL")
      w340 = u8 2 items=["Fully Auto", "OPEN", "CLOSED"] ("Shutter Mode")
      w341 = u16 0 items=["Cooler OFF", "Cooler ON"] ("Cooler ON/OFF")
      w344 = u8 0 items=["Electron Multiplying", "Conventional"] ("EM Mode")
      w345 = u8 0 items=["1 MHz", "10 MHz", "20 MHz", "30 MHz"] ("Readout Rate")
      w346 = u8 0 items=["Gain 1", "Gain 2"] ("Pre-amp gain")
      w347 = u8 3 items=["0.6", "1.13", "2.2", "4.33"] ("Vertical Shift Speed")
      w348 = u8 4 items=["Full Vertical Binning", "Multi-Track", "Random-track", "Single-Track", "Image"] ("Read Mode")
      w321 = u8 0 items=["Internal", "External"] ("Trigger")
      w349 = u8 1 items=["N/A", "Single", "Accumulate", "Kinetic", "Fast Kinetic"] ("Acquisition Mode")
      w350 = u16 1 ("Vertical Binning")
      w351 = u16 1024 ("Final Line")
      w352 = u16 1 ("Initial Line")
      n139 = Bundle(u32 1985280, u32 1985280) -> (w335:cluster{u32, u32})  [unwired: 1 in]
      n140 = local write "% Acquired"(0.0 ("% Acquired")) -> ()
      n141 = local write "Exposing"(FALSE ("Exposing")) -> ()
      n142 = local write "Exposições realizadas"(u8 0 ("Exposições realizadas")) -> ()
      n143 = local write "Initial Line"(w352) -> ()
      n144 = local write "Initial Cloumn"(w352) -> ()
      n145 = local write "Final Line"(w351) -> ()
      n146 = local write "Final Column"(w351) -> ()
      n147 = local write "Vertical Binning"(w350) -> ()
      n148 = local write "Horizontal Binning"(w350) -> ()
      n149 = local write "Acquisition Mode"(w349) -> ()
      n150 = local write "Stop Button"(w337) -> ()
      n151 = local write "Initialization"(w337) -> ()
      n152 = local write "Vertical Clock  Amplitude"(w322) -> ()
      n153 = Build Array(w335) -> (w336:cluster{u32, u32}[])
      n154 = local write "Temperature"(i16 20 ("Temperature")) -> ()
      n155 = property on="Readout Rate" class="Ring (strict)"("Strings []"=string[] ["30 MHz", "20 MHz", "10 MHz", "  1 MHz"]) -> ()  [unwired: 2 in, 2 out]
      n156 = property on="Initialization" class="Bool (strict)"("Colors [4]"=w336) -> ()  [unwired: 2 in, 2 out]
      n157 = property on="Temperature" class="DigNum (strict)"("NumText.BGColor"=w331) -> ()  [unwired: 2 in, 2 out]
      n158 = property on="Temperature" class="DigNum (strict)"("NumText.BG Color"=w331) -> ()  [unwired: 2 in, 2 out]
      n159 = local write "Readout Time (ms)"(39.38645333333 ("Readout Time")) -> ()
      n160 = local write "Kinetic Series Length"(u32 1 ("Kinetic Series Length")) -> ()
      n161 = local write "Kinetic Cycle Time"(u32 0 ("Kinetic Cycle Time")) -> ()
      n162 = local write "Number of Accum."(u32 1 ("Number of Accum.")) -> ()
      n163 = local write "Frame Transfer"(FALSE ("Frame Transfer")) -> ()
      n164 = local write "Read Mode"(w348) -> ()
      n165 = local write "Vertical Shift Speed"(w347) -> ()
      n166 = local write "Pre-amp gain"(w346) -> ()
      n167 = local write "Readout Rate"(w345) -> ()
      n168 = local write "EM Mode"(w344) -> ()
      n169 = local write "EM Gain"(u16 2 ("EM Gain")) -> ()
      n170 = local write "Set temperature"(i8 20 ("Set temperature")) -> ()
      n171 = local write "Cooler ON/OFF"(w341) -> ()
      n172 = local write "Shutter Mode"(w340) -> ()
      n173 = local write "Shutter TTL"(w339) -> ()
      n174 = local write "Time to close shutter"(w338) -> ()
      n175 = local write "Time to open shutter"(w338) -> ()
      n176 = local write "Exposure Time"(u32 0 ("Exposure Time")) -> ()
      n177 = local write "# Images"(u32 1 ("# Images")) -> ()
      n178 = local write "Trigger"(w321) -> ()
    }
  }
